vi "Render.vi"(8 "error in (no error)":errorcluster, 10 "String in":string, 11 "Strikethrough in":refnum<class "Strikethrough.lvclass">) -> (0 "error out":errorcluster, 2 "String out":string, 3 "Strikethrough out":refnum<class "Strikethrough.lvclass">)   [LabVIEW 2021, in "LvMarkdown.lvlib" / "Strikethrough.lvclass"]
uses:
  Strikethrough.lvclass
  Strikethrough.lvclass/Strikethrough.ctl
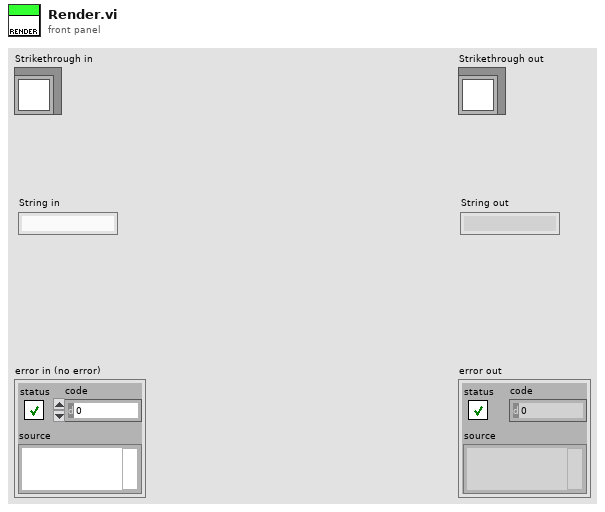
[diagram p1: front panel]
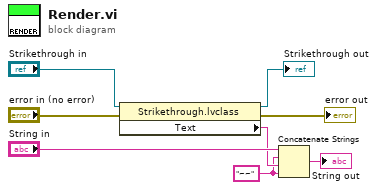
[diagram p0: block diagram]
diagram:
  w2 = "~~" ("string")
  n1 = property class="Strikethrough.lvclass"(reference="Strikethrough in", error in="error in (no error)") -> (reference out=→"Strikethrough out":refnum<class "Strikethrough.lvclass">, error out=→"error out":errorcluster, "Text"=w3:string)
  n2 = Concatenate Strings("String in", w2, w3, w2) -> (→"String out":string)
